vi "Load Asked Questions from Disk.vi"(8 "error in (no error)":errorcluster, 11 "Controller in":refnum<class "Controller.lvclass">) -> (0 "error out":errorcluster, 3 "Controller out":refnum<class "Controller.lvclass">)   [LabVIEW 2024, in "Controller.lvlib" / "Controller.lvclass"]
uses:
  Controller.lvclass
  Controller.lvclass/Controller.ctl
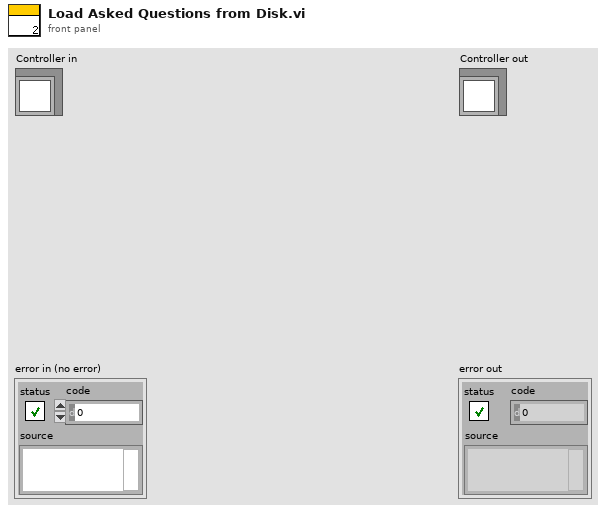
[diagram p1: front panel]
types:
  T1 = enum16{"open", "replace", "create", "open or create", "replace or create", "replace or create with confirmation"}
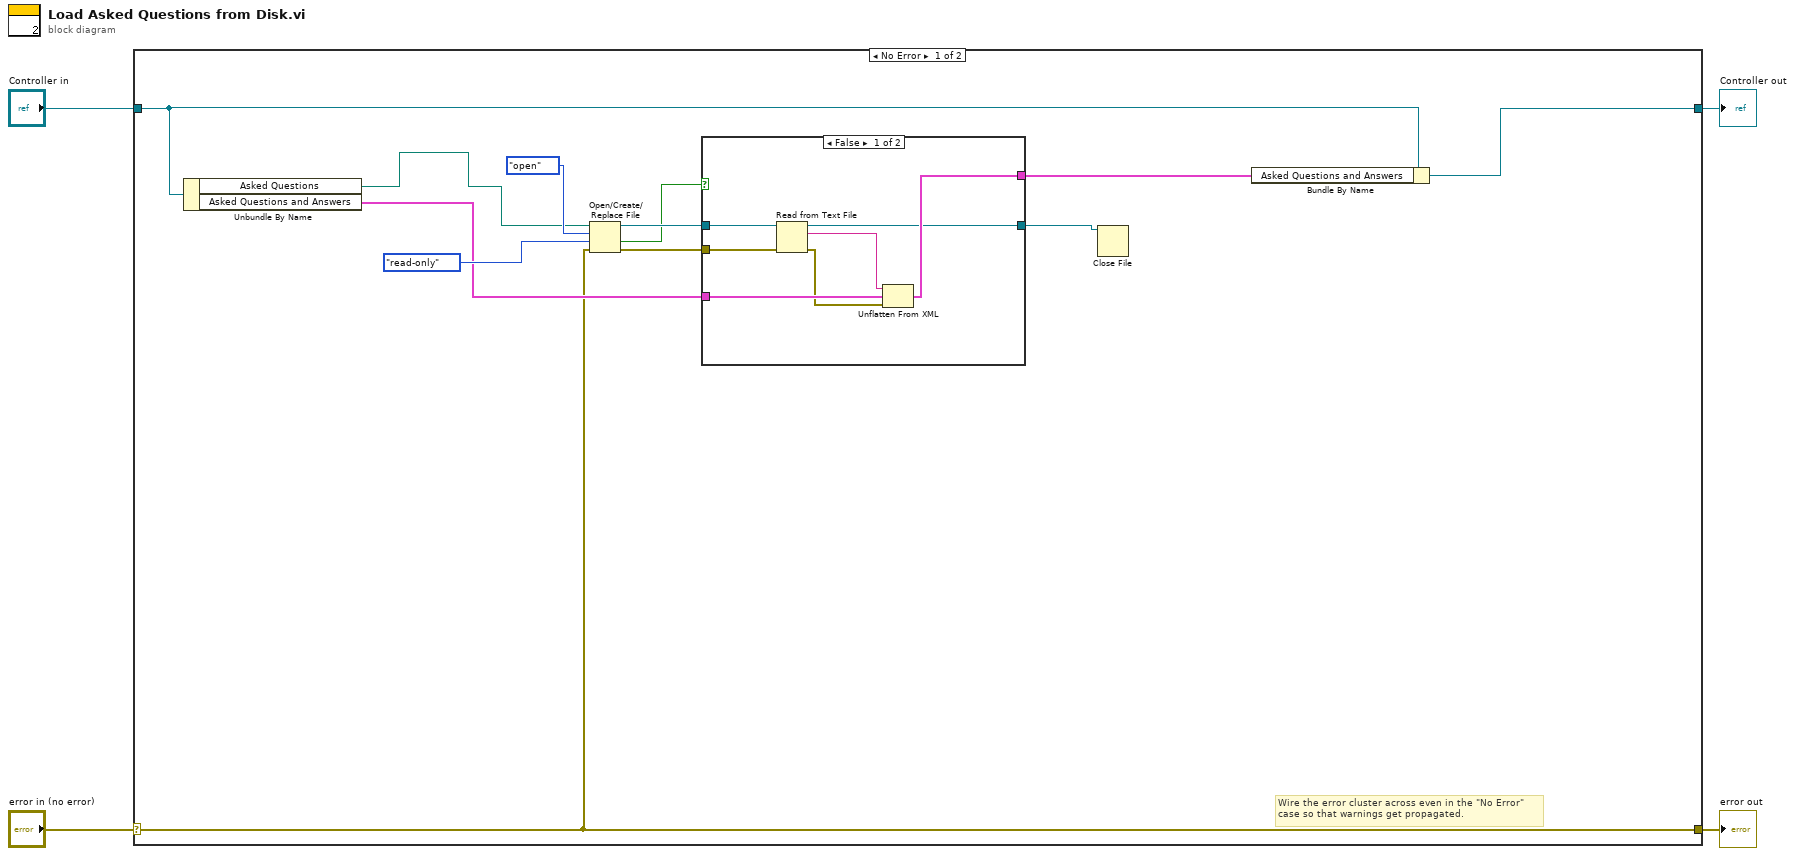
[diagram p0: block diagram]
diagram:
  n1 = case shown="No Error" "error in (no error)" {
    selector: "error in (no error)" -> [w6 w26]
    tunnel: [w6 w26] -> w3
    tunnel: [w16 w25] -> w1
    tunnel: "Controller in" -> [w10 w25]
    frame No Error {
      # "Wire the error cluster across even in the \"No Error\"\ncase so that warnings get propagated."
      n2 = Unbundle By Name(w10) -> ("Asked Questions"=w5:path, "Asked Questions and Answers"=w8:cluster{"String":string, "String":string}[])
      n3 = Open/Create/Replace File(file path (use dialog)=w5, error in=w6, operation (0:open)=T1."open", access (0:read/write)=enum16{"read/write", "read-only", "write-only"}."read-only") -> (refnum out=w12:refnum<file>, cancelled=w11:bool, error out=w13:errorcluster)  [unwired: 2 in]
      n4 = case shown="False" w11 {
        tunnel: w8 -> [w23 _]
        tunnel: w13 -> [w22 _]
        tunnel: w12 -> [w20 w24]
        tunnel: [w19 _] -> w7
        tunnel: [w17 w24] -> w9
        frame False {
          n5 = Read from Text File(file (use dialog)=w20, error in=w22) -> (refnum out=w17:refnum<file>, text=w21:string, error out=w18:errorcluster)  [unwired: 2 in, 1 out]
          n6 = Unflatten From XML(xml string=w21, type=w23, error in (no error)=w18) -> (value=w19:cluster{"String":string, "String":string}[])  [unwired: 1 out]
        }
        frame True {
        }
      }
      n7 = Close File(refnum=w9) -> ()  [unwired: 1 in, 2 out]
      n8 = Bundle By Name(cluster=w10, "Asked Questions and Answers"=w7) -> (w16:refnum<class "Controller.lvclass">)
    }
    frame Error {
    }
  }
  "error out" <- w3
  "Controller out" <- w1
